vi "S2C_Shared_Proc_ManageError.vi"(5 "Local?":bool, 7 "Process":string, 8 "Error In":errorcluster, 11 "Data":variant) -> (0 "Error Out":errorcluster)   [LabVIEW 2024]
doc: "Write an error to file, displays the error to the user, and exits the application if warranted."
uses:
  <vilib>/Utility/error.llb/DialogType.ctl
  <vilib>/Utility/error.llb/Trim Whitespace One-Sided.vi
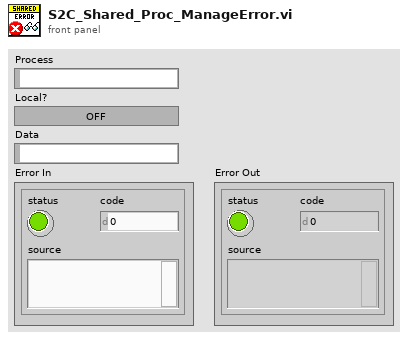
[diagram p1: front panel]
types:
  T1 = typedef "DialogType.ctl" = u16
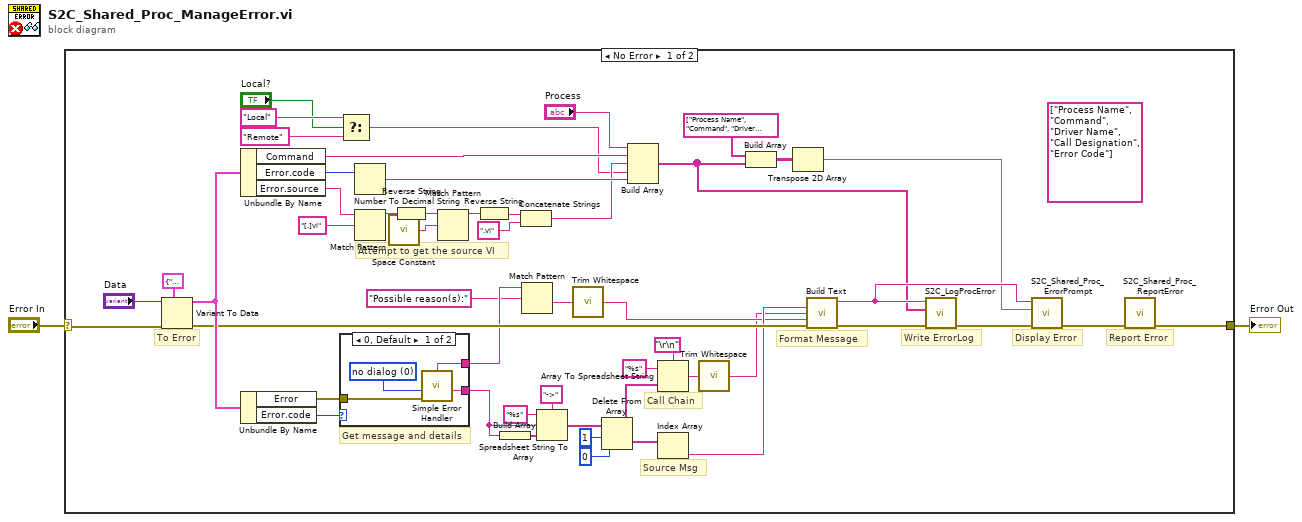
[diagram p0: block diagram]
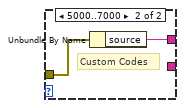
[diagram p2: hidden frame]
diagram:
  n1 = case shown="No Error" "Error In" {
    selector: "Error In" -> [w3 w60]
    tunnel: [w4 w60] -> w1
    frame No Error {
      (unwired) string[] ["Process Name", "Command", "Driver Name", "Call Designation", "Error Code"]
      # "Report Error"
      # "Source Msg"
      # "Call Chain"
      # "Format Message"
      # "Attempt to get the source VI"
      # "Get message and details"
      # "To Error"
      # "Display Error"
      # "Write ErrorLog"
      n2 = Variant To Data(error in=w3, type=cluster{"Command":string, "Error":errorcluster} {"Command"="", "Error"={"status"=FALSE, "code"=0, "source"=""}}, Variant="Data") -> (data=w50:cluster{"Command":string, "Error":errorcluster}, error out=w24:errorcluster)
      n3 = Unbundle By Name(w50) -> ("Command"=w35:string, "Error.code"=w34:i32, "Error.source"=w33:string)
      n4 = Unbundle By Name(w50) -> ("Error"=w29:errorcluster, "Error.code"=w30:i32)
      n5 = case shown="0, Default" w30 {
        tunnel: w29 -> [w57 w59]
        tunnel: [w55 w58] -> w13
        tunnel: [w54 _] -> w25
        frame 0, Default {
          w56 = T1 0 items=["no dialog", "OK message", "continue or stop message", "OK message + warnings", "continue/stop + warnings"] ("type of dialog (OK msg:1)")
          n6 = call <vilib>:"Simple Error Handler.vi"("type of dialog (OK msg:1)"=w56, "error in (no error)"=w57) -> ("source out"=w54:string, "message"=w55:string)  [unwired: 3 in, 3 out]
        }
        frame 5000..7000 {
          # "Custom Codes"
          n7 = Unbundle By Name(w59) -> ("source"=w58:string)
        }
      }
      n8 = Select(t="Local", s="Local?", f="Remote") -> (s? t:f=w31:string)
      n9 = Number To Decimal String(number=w34) -> (decimal integer string=w42:string)  [unwired: 1 in]
      n10 = Match Pattern(string=w33, regular expression="[.]vi") -> (before substring=w47:string)  [unwired: 1 in, 3 out]
      n11 = call <vilib>:"Space Constant.vi"() -> ("String"=w48:string)
      n12 = Reverse String(1:w47) -> (0:w46:string)
      n13 = Match Pattern(string=w46, regular expression=w48) -> (before substring=w45:string)  [unwired: 1 in, 3 out]
      n14 = Reverse String(1:w45) -> (0:w44:string)
      n15 = Build Array(w25) -> (w27:string[])
      n16 = Concatenate Strings(w44, ".vi" ("string")) -> (w32:string)
      n17 = Match Pattern(string=w13, regular expression="Possible reason(s):") -> (after substring=w10:string)  [unwired: 1 in, 3 out]
      n18 = Spreadsheet String To Array(delimiter (Tab)="->", format string="%s", spreadsheet string=w25, array type (2D Dbl)=w27) -> (array=w22:string[])
      n19 = call <vilib>:"Trim Whitespace.vi"("string"=w10) -> ("trimmed string"=w9:string)  [unwired: 1 in]
      n20 = Delete From Array(array=w22, length=1, index=0) -> (deleted portion=w19:string[], array with subset deleted=w17:string[])
      n21 = Build Array("Process", w35, w32, w31, w42) -> (w6:string[])
      n22 = Array To Spreadsheet String(delimiter (Tab)="\r\n", array=w17, 3:"%s" ("format string")) -> (spreadsheet string=w14:string)
      n23 = Index Array(array=w19) -> (element=w18:string)  [unwired: 1 in]
      n24 = call <vilib>:"Trim Whitespace.vi"("string"=w14) -> ("trimmed string"=w8:string)  [unwired: 1 in]
      n25 = Build Array(string[] ["Process Name", "Command", "Driver Name", "Call Designation", "Error Code"], w6) -> (w41:string[][])
      n26 = Transpose 2D Array(2D array=w41) -> (transposed array=w7:string[][])
      n27 = call "Build Text"("Source"=w18, "Chain"=w8, "Reason"=w9, "error in (no error)"=w24) -> ("Result"=w11:string, "error out"=w23:errorcluster)  [unwired: 10 in]
      n28 = call "S2C_LogProcError.vi"("Error In"=w23, "Error Details"=w6, "Error Msg"=w11) -> ("Error Out"=w53:errorcluster)  [unwired: 8 in]
      n29 = call "S2C_Shared_Proc_ErrorPrompt.vi"("Error In"=w53, "Parameters"=w7, "ErrMsgIn"=w11) -> ("Error Out"=w5:errorcluster)  [unwired: 8 in]
      n30 = call "S2C_Shared_Proc_ReportError.vi"("Error In"=w5) -> ("Error Out"=w4:errorcluster)  [unwired: 10 in]
    }
    frame Error {
    }
  }
  "Error Out" <- w1
